vi "Ramp Rate Updated.vi"(8 "error in (no error)":errorcluster, 10 "Temperature Ramp Rate":dbl) -> (0 "error out":errorcluster)   [LabVIEW 2015, in "Thermal Chamber Controller_DQMH.lvlib"]
doc: "Broadcast to any VI registered to listen to Thermal Chamber Controller's broadcast events that the Ramp Rate was updated.\n_____\nCreated using Delacor QMH Event Scripter 1.0.0.50.\n____\nDelacor QMH Thermal Chamber Examples 4.0.0.21\nCopyright (c) 2018, Delacor"
uses:
  Thermal Chamber Controller_DQMH.lvlib
  Update Ramp Rate Argument--cluster.ctl
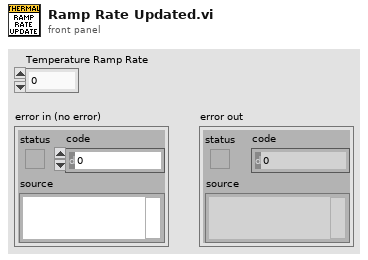
[diagram p1: front panel]
types:
  T1 = typedef "Thermal Chamber Controller_DQMH.lvlib/Update Ramp Rate Argument--cluster.ctl" = cluster{"Temperature Ramp Rate":dbl}
  T2 = typedef "Thermal Chamber Controller_DQMH.lvlib/Broadcast Events--cluster.ctl" = cluster{"Module Did Init":refnum<user-event>, "Status Updated":refnum<user-event>, "Error Reported":refnum<user-event>, "Module Did Stop":refnum<user-event>, "Update Module Execution Status":refnum<user-event>, "Set Point Updated":refnum<user-event>, "Ramp Rate Updated":refnum<user-event>, "Heater State Updated":refnum<user-event>, "Chamber Status Updated":refnum<user-event>}
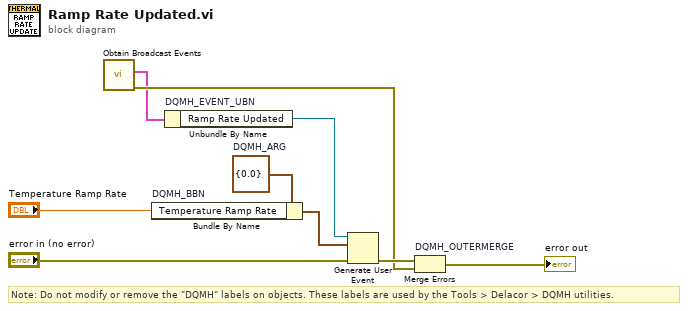
[diagram p0: block diagram]
diagram:
  w4 = T1 {"Temperature Ramp Rate"=0.0}  # DQMH_ARG
  # "Note: Do not modify or remove the \"DQMH\" labels on objects. These labels are used by the Tools > Delacor > DQMH utilities."
  n1 = call "Obtain Broadcast Events.vi"() -> ("error out"=w2:errorcluster, "Thermal Chamber Controller_DQMH Broadcast Events"=w1:T2)  [unwired: 10 in]
  n2 = Bundle By Name "DQMH_BBN"(cluster=w4, "Temperature Ramp Rate"="Temperature Ramp Rate") -> (w6:T1)
  n3 = Unbundle By Name "DQMH_EVENT_UBN"(w1) -> ("Ramp Rate Updated"=w5:refnum<user-event>)
  n4 = Generate User Event(user event=w5, event data cluster=w6, error in="error in (no error)") -> (error out=w7:errorcluster)  [unwired: 1 in, 1 out]
  n5 = Merge Errors "DQMH_OUTERMERGE"(w7, w2) -> (→"error out":errorcluster)
